vi "ToggleByRoomName.vi"(0 "reference in":refnum<class "HeatingSystem.lvclass">, 2 "RoomName":string, 5 "Error In":errorcluster) -> (14 "reference out":refnum<class "HeatingSystem.lvclass">, 19 "Error Out":errorcluster)   [LabVIEW 2024, in "HeatingSystem.lvclass"]
uses:
  HeatingSystem.lvclass
  HeatingSystem.lvclass/HeatingSystem.ctl
  Devices/Air Conditioner_class/Air Conditioner.lvclass
  House/Room_class/Room.lvclass
panel:
  # "Connector Pane"
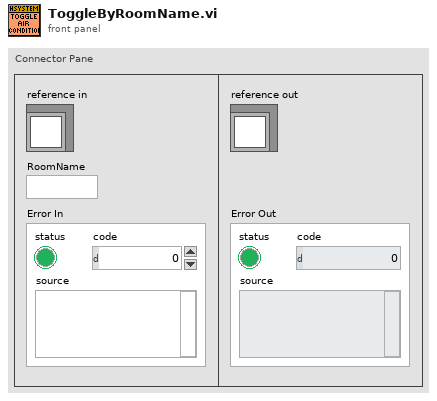
[diagram p1: front panel]
types:
  T1 = typedef "HeatingSystem.lvclass/ObjectAttributes.ctl" = cluster{"Rooms":T2}
  T2 = typedef "Rooms Map.ctl" = map{string, refnum<class "Room.lvclass">}
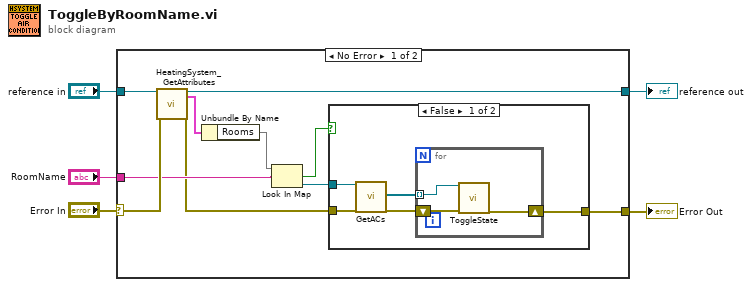
[diagram p0: block diagram]
diagram:
  n1 = case shown="No Error" "Error In" {
    selector: "Error In" -> [w15 w26]
    tunnel: [w6 w26] -> w4
    tunnel: [w12 w25] -> w2
    tunnel: "reference in" -> [w13 w25]
    tunnel: "RoomName" -> [w10 _]
    frame No Error {
      n2 = call "HeatingSystem_GetAttributes.vi"("reference in"=w13, "Error In"=w15) -> ("reference out"=w12:refnum<class "HeatingSystem.lvclass">, "Data"=w14:T1, "Error Out"=w7:errorcluster)  [unwired: 14 in, 1 out]
      n3 = Unbundle By Name(w14) -> ("Rooms"=w11:T2)
      n4 = Look In Map(map=w11, key=w10) -> (key not found?=w9:bool, value=w8:refnum<class "Room.lvclass">)  [unwired: 1 in]
      n5 = case shown="False" w9 {
        tunnel: w8 -> [w20 _]
        tunnel: w7 -> [w17 w24]
        tunnel: [w16 w24] -> w6
        frame False {
          n6 = call-dynamic "GetACs.vi"("reference in"=w20, "Error In"=w17) -> ("ACs"=w18:refnum<class "Air Conditioner.lvclass">[], "Error Out"=w19:errorcluster)  [unwired: 15 in, 1 out]
          n7 = for {
            tunnel: w18 -> [w22] mode=indexing
            shift-right: [w21] -> w16
            shift-left: w19 -> [w23]
            n8 = call "ToggleState.vi"("reference in"=w22, "Error In"=w23) -> ("Error Out"=w21:errorcluster)  [unwired: 16 in, 1 out]
          }
        }
        frame True {
        }
      }
    }
    frame Error {
    }
  }
  "Error Out" <- w4
  "reference out" <- w2
